vi "Dequeue element.vi"(8 "error in (no error)":errorcluster) -> (0 "error out":errorcluster, 3 "Message":T1)   [LabVIEW 2018, in "Template Module.lvlib"]
doc: "Dequeues element"
uses:
  Template Module.lvlib
  ctl/Message--enum.ctl
  ctl/State--enum.ctl
  ctl/Queue action--enum.ctl
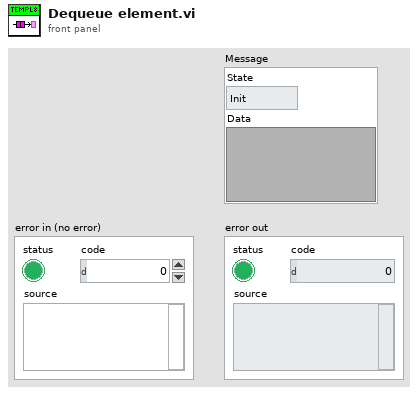
[diagram p1: front panel]
types:
  T1 = typedef "Template Module.lvlib/Message--enum.ctl" = cluster{"State":T2, "Data":variant}
  T2 = typedef "Template Module.lvlib/State--enum.ctl" = enum16{"Init", "Error", "Close"}
  T3 = typedef "Template Module.lvlib/Queue action--enum.ctl" = enum16{"Create", "Get", "Destroy"}
  T4 = typedef "Message--enum.ctl" = cluster{"State":T5, "Data":variant}
  T5 = typedef "State--enum.ctl" = enum16{"Init", "Error", "Close"}
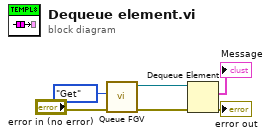
[diagram p0: block diagram]
diagram:
  n1 = call "Queue FGV.vi"("error in"="error in (no error)", "Queue Action"=Queue_action--enum."Get") -> ("error out"=w1:errorcluster, "Queue reference"=w2:refnum<queue>)  [unwired: 8 in]
  n2 = Dequeue Element(queue=w2, error in (no error)=w1) -> (element=→"Message":T4, error out=→"error out":errorcluster)  [unwired: 1 in, 2 out]
